vi "Form_HistoricalDataQuery.vi"() -> ()   [LabVIEW 2018]
panel:
  in  "表格/图形":enum32{"table", "graph"}(radio)
  in  "导出曲线":bool
  in  "查询数据":bool
  in  "导出数据":bool
  in  "Ring_查询仪表":u16(ring) caption="查询仪表" items=["电参数1", "电参数2", "温度"]
  in  "Ring_查询月份":u16(ring) caption="查询年月" items=["电参数1", "电参数2", "温度"]
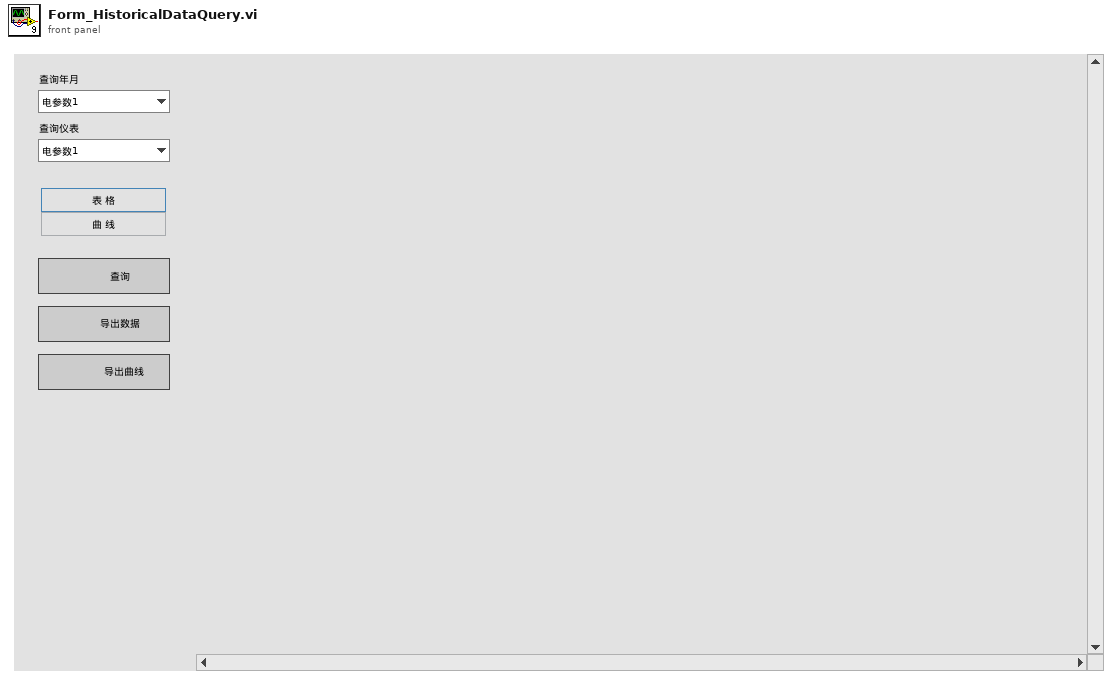
[diagram p1: front panel]
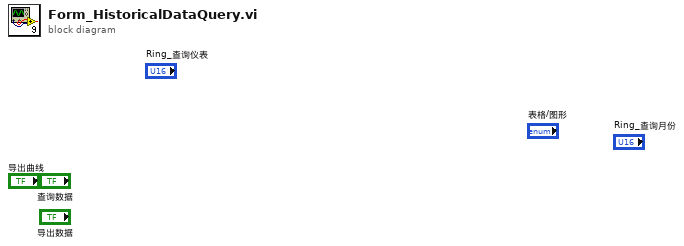
[diagram p0: block diagram]
diagram:
